vi "PythonCaller.vi"() -> ()   [LabVIEW 2019]
uses:
  target -- cluster.ctl
  e185c1da-ac2d-4450-977a-4885e821bdf8.vi
  <vilib>/JDP Science/JSONtext/Variant to JSON Text.vi
  <vilib>/JDP Science/JSONtext/LVClass Serializer/JSONtext LVClass Serializer.lvclass
panel:
  in  "Connect":bool
  in  "Tab Control":T1(tab)
  in  "Enable Cmd":bool
  in  "Temperature Setpoint":dbl format="%.1g"
  in  "RunCycle":bool
  in  "nb_loops":u8=1 min=1 max=50 step=1
  in  "Launch GUI":bool
  out "error":errorcluster
  out "return value":string
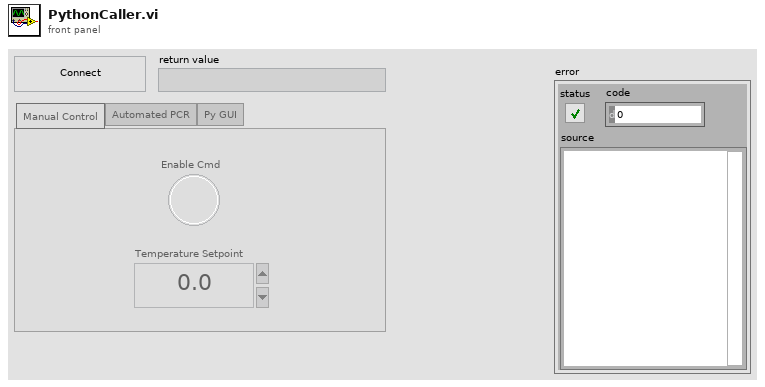
[diagram p1: front panel]
types:
  T1 = enum32{"Manual Control", "Automated PCR", "Py GUI"}
  T2 = enum8{"Enabled", "Disabled", "Disabled and Grayed Out"}
  T3 = cluster{"appName":string, "remoteName":string, "mqtt-python":path, "Python session":refnum<k35>}
  T4 = typedef "target -- cluster.ctl" = cluster{"enabled":bool, "setpoint":dbl, "responseURI":string}
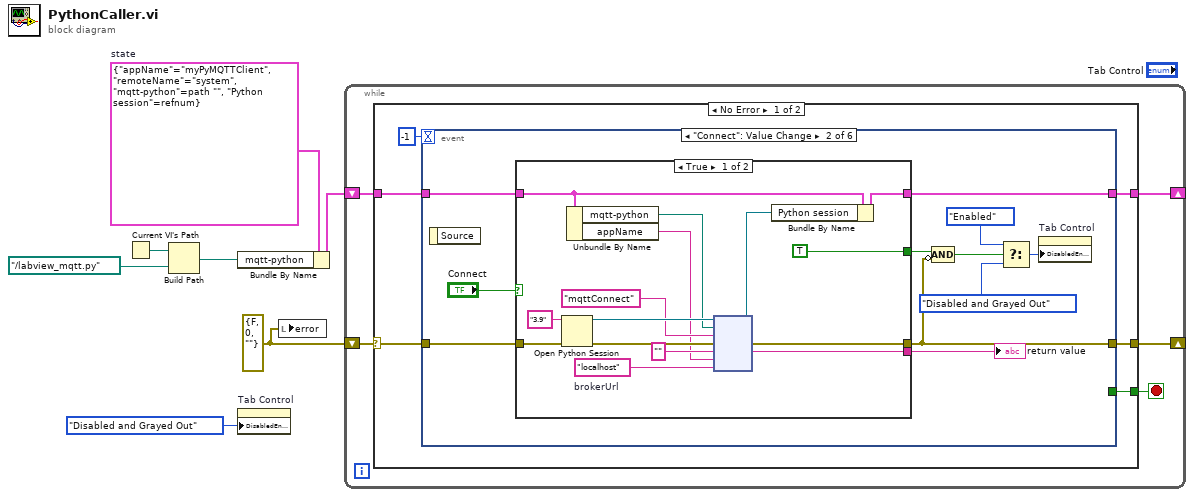
[diagram p0: block diagram]
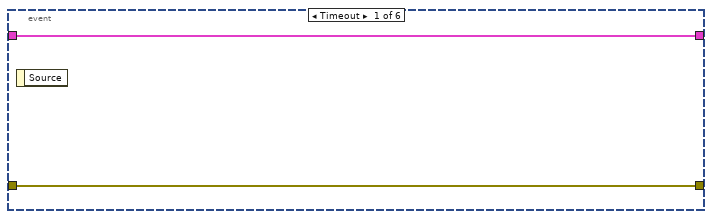
[diagram p2: hidden frame]
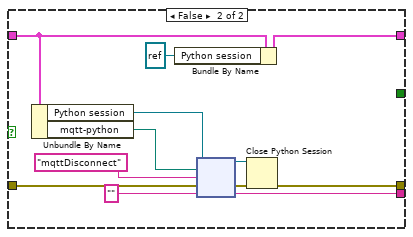
[diagram p3: hidden frame]
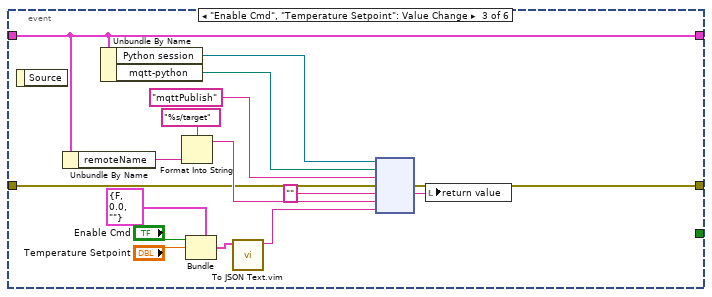
[diagram p4: hidden frame]
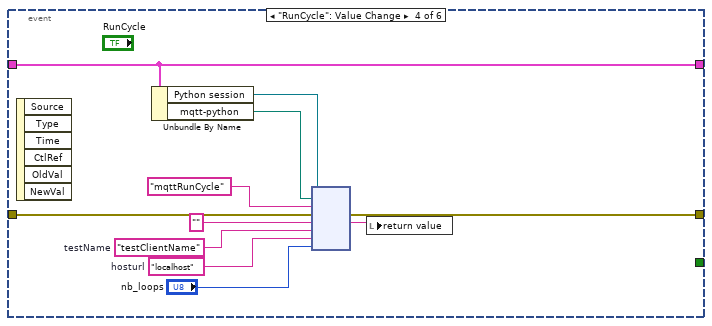
[diagram p5: hidden frame]
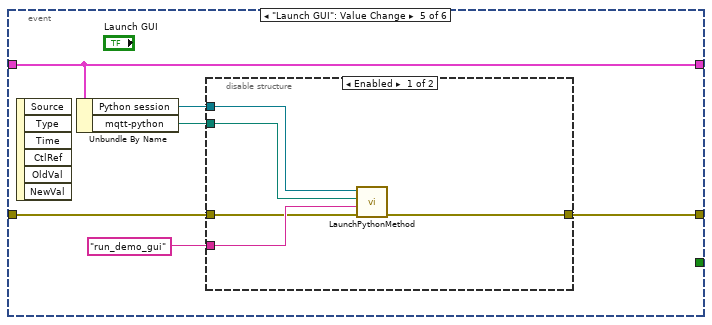
[diagram p6: hidden frame]
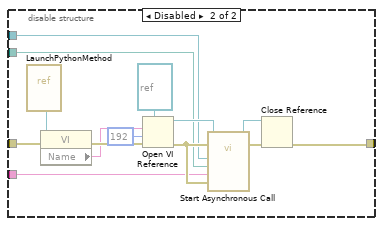
[diagram p7: hidden frame]
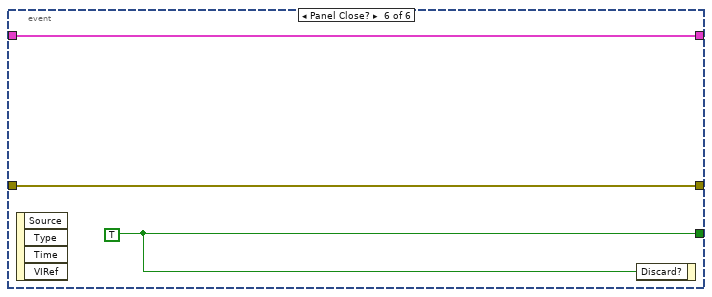
[diagram p8: hidden frame]
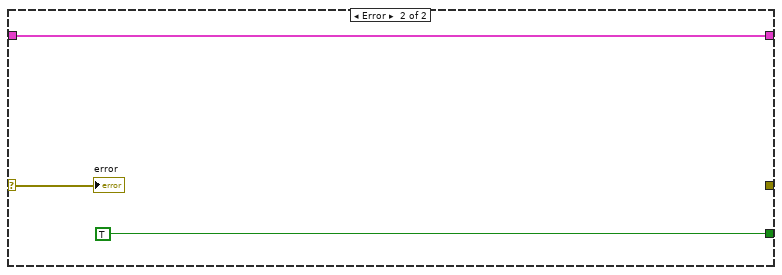
[diagram p9: hidden frame]
diagram:
  w2 = errorcluster {"status"=FALSE, "code"=0, "source"=""} ("error IO")
  w7 = T3 {"appName"="myPyMQTTClient", "remoteName"="system", "mqtt-python"=path "", "Python session"=refnum}  # state
  n1 = Current VI's Path() -> (path=w5:path)
  n2 = Build Path(base path=w5, name or relative path=path "../labview_mqtt.py") -> (appended path=w3:path)
  n3 = Bundle By Name(cluster=w7, "mqtt-python"=w3) -> (w6:T3)
  n4 = property on="Tab Control" class="TabCtl (strict)"("DisabledEnum"=T2."Disabled and Grayed Out" ("Disabled")) -> ()  [unwired: 2 in, 2 out]
  n5 = local write "error"(w2) -> ()
  n6 = while {
    shift-right: [w12] -> _
    shift-left: w2 -> [w10]
    shift-right: [w8] -> _
    shift-left: w6 -> [w9]
    stop <- w11 stop-if-true
    n7 = case shown="No Error" w10 {
      selector: w10 -> [w15 w114]
      tunnel: [w18 _] -> w12
      tunnel: [w16 TRUE] -> w11
      tunnel: w9 -> [w14 w116]
      tunnel: [w13 w116] -> w8
      frame No Error {
        n8 = event shown="[1] \"Connect\": Value Change" {
          selector: _ -> [_ _ _ _ _ _]
          dyn-events: _ -> [_ _ _ _ _ _]
          timeout: -1 -> [_ _ _ _ _ _]
          tunnel: w15 -> [w19 w28 w61 w76 w88 w112]
          tunnel: [w19 w22 w62 w77 w87 w112] -> w18
          tunnel: [_ _ _ _ _ w113] -> w16
          tunnel: w14 -> [w20 w29 w70 w82 w91 w111]
          tunnel: [w20 w30 w70 w82 w91 w111] -> w13
          event Timeout {
            n9 = event-data() -> ()  [unwired: 1 in, 1 out]
          }
          event "Connect": Value Change {
            n10 = event-data() -> ()  [unwired: 1 in, 1 out]
            n11 = case shown="True" "Connect" {
              tunnel: [w41 w57] -> w31
              tunnel: [w38 w55] -> w30
              tunnel: w29 -> [w37 w54]
              tunnel: [w35 w47] -> w22
              tunnel: w28 -> [w34 w53]
              tunnel: [TRUE _] -> w23
              frame True {
                w40 = "localhost"  # brokerUrl
                n12 = Open Python Session(python version="3.9" ("Python version"), 3:w34) -> (session out=w45:refnum<k35>, error out=w44:errorcluster)  [unwired: 1 in]
                n13 = Unbundle By Name(w37) -> ("mqtt-python"=w39:path, "appName"=w36:string)
                n14 = node(w45, w39, "mqttConnect" ("Python version"), w44, "" ("Python version"), w36, w40) -> (w33:refnum<k35>, w35:errorcluster, w41:string)  [unwired: 2 in, 2 out]
                n15 = Bundle By Name(cluster=w37, "Python session"=w33) -> (w38:T3)
              }
              frame False {
                n16 = Unbundle By Name(w54) -> ("Python session"=w51:refnum<k35>, "mqtt-python"=w56:path)
                n17 = Bundle By Name(cluster=w54, "Python session"=refnum<k35> refnum) -> (w55:T3)
                n18 = node(w51, w56, "mqttDisconnect" ("Python version"), w53, "" ("Python version")) -> (w49:refnum<k35>, w48:errorcluster, w57:string)  [unwired: 2 out]
                n19 = Close Python Session(session in=w49, error in=w48) -> (11:w47:errorcluster)
              }
            }
            "return value" <- w31
            n20 = Compound Arithmetic op=AND(w23, invert w22) -> (w21:bool)
            n21 = Select(t=T2."Enabled" ("Disabled"), s=w21, f=T2."Disabled and Grayed Out" ("Disabled")) -> (s? t:f=w26:T2)
            n22 = property on="Tab Control" class="TabCtl (strict)"("DisabledEnum"=w26) -> ()  [unwired: 2 in, 2 out]
          }
          event "Enable Cmd", "Temperature Setpoint": Value Change {
            n23 = event-data() -> ()  [unwired: 1 in, 1 out]
            n24 = Unbundle By Name(w70) -> ("remoteName"=w69:string)
            n25 = Unbundle By Name(w70) -> ("Python session"=w59:refnum<k35>, "mqtt-python"=w72:path)
            n26 = Format Into String(format string="%s/target", w69) -> (resulting string=w67:string)  [unwired: 2 in, 1 out]
            n27 = Bundle(cluster=T4 {"enabled"=FALSE, "setpoint"=0.0, "responseURI"=""} ("target"), "enabled"="Enable Cmd", "setpoint"="Temperature Setpoint") -> (w64:T4)  [unwired: 1 in]
            n28 = call "To JSON Text.vim"("Anything"=w64) -> ("<JSON>"=w63:string)  [unwired: 9 in, 1 out]
            n29 = node(w59, w72, "mqttPublish" ("Python version"), w61, "" ("Python version"), w67, w63) -> (w62:errorcluster, w71:string)  [unwired: 2 in, 3 out]
            n30 = local write "return value"(w71) -> ()
          }
          event "RunCycle": Value Change {
            w79 = "localhost"  # hosturl
            w80 = "testClientName"  # testName
            n31 = event-data() -> ()  [unwired: 1 in, 6 out]
            n32 = Unbundle By Name(w82) -> ("Python session"=w78:refnum<k35>, "mqtt-python"=w75:path)
            n33 = node(w78, w75, "mqttRunCycle" ("Python version"), w76, "" ("Python version"), w80, w79, "nb_loops") -> (w77:errorcluster, w83:string)  [unwired: 3 in, 3 out]
            n34 = local write "return value"(w83) -> ()
          }
          event "Launch GUI": Value Change {
            n35 = event-data() -> ()  [unwired: 1 in, 6 out]
            n36 = Unbundle By Name(w91) -> ("Python session"=w90:refnum<k35>, "mqtt-python"=w89:path)
            n37 = disable-structure shown="Enabled" {
              disable-tunnel: w90 -> [w96 w99]
              disable-tunnel: w89 -> [w95 w98]
              disable-tunnel: "run_demo_gui" ("Python version") -> [w94 w100]
              disable-tunnel: w88 -> [w93 w109]
              disable-tunnel: [w92 w102] -> w87
              frame Enabled {
                n38 = call "LaunchPythonMethod.vi"("Error In"=w93, "Method Name"=w94, "Python Module Path"=w95, "Python session"=w96) -> ("Error Out"=w92:errorcluster)  [unwired: 7 in]
              }
              frame Disabled {
                n39 = vi-ref "LaunchPythonMethod.vi"() -> (w108:refnum<vi>)
                n40 = property class="VI"(reference=w108, error in=w109) -> (error out=w110:errorcluster, "Name"=w107:string)  [unwired: 1 out]
                n41 = Open VI Reference(type specifier VI Refnum (for type only)=refnum<vi> refnum, vi path=w107, options=192, error in (no error)=w110) -> (vi reference=w105:refnum<vi>, error out=w101:errorcluster)  [unwired: 2 in]
                n42 = call-by-ref "Start Asynchronous Call"(reference=w105, error in=w101, "Error In"=w101, "Method Name"=w100, "Python Module Path"=w98, "Python session"=w99) -> (reference out=w103:refnum<vi>, error out=w104:errorcluster)  [unwired: 7 in, 1 out]
                n43 = Close Reference(reference=w103, error in (no error)=w104) -> (error out=w102:errorcluster)
              }
            }
          }
          event Panel Close? {
            w113 = TRUE
            n44 = event-data() -> ()  [unwired: 1 in, 4 out]
            n45 = event-data("Discard?"=w113) -> ()  [unwired: 1 in, 1 out]
          }
        }
      }
      frame Error {
        "error" <- w114
      }
    }
  }
